vi "getKeithleyScriptPath.vi"(8 "error in (no error)":errorcluster, 11 "FileSystem in":refnum<class "FileSystem.lvclass">) -> (0 "error out":errorcluster, 2 "keithleyScriptPath":path, 3 "FileSystem out":refnum<class "FileSystem.lvclass">)   [LabVIEW 2011, in "Tools.lvlib" / "Filing.lvlib" / "FileSystem.lvclass"]
uses:
  FileSystem.lvclass
  FileSystem.lvclass/FileSystem.ctl
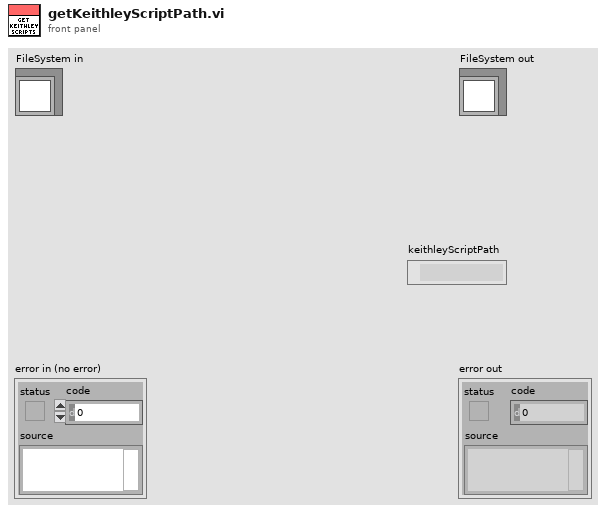
[diagram p1: front panel]
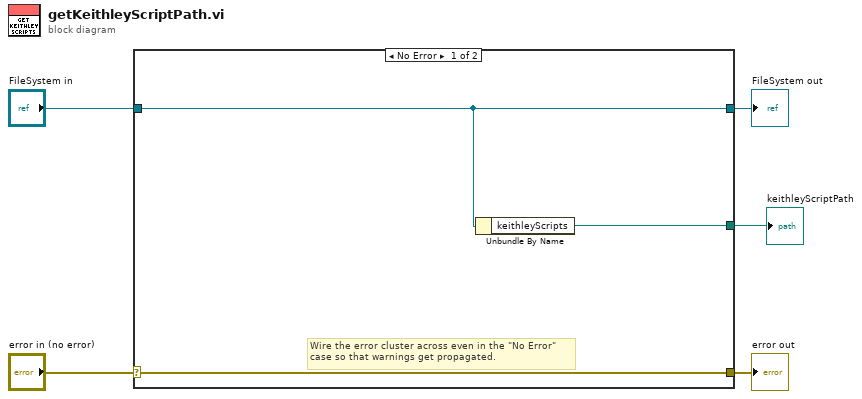
[diagram p0: block diagram]
diagram:
  n1 = case shown="No Error" "error in (no error)" {
    selector: "error in (no error)" -> [w8 w10]
    tunnel: [w8 w10] -> w4
    tunnel: [w7 w9] -> w2
    tunnel: "FileSystem in" -> [w7 w9]
    tunnel: [w6 _] -> w1
    frame No Error {
      # "Wire the error cluster across even in the \"No Error\"\ncase so that warnings get propagated."
      n2 = Unbundle By Name(w7) -> ("keithleyScripts"=w6:path)
    }
    frame Error {
    }
  }
  "error out" <- w4
  "FileSystem out" <- w2
  "keithleyScriptPath" <- w1
